vi "cache tag indices.vi"(8 "error in":errorcluster, 9 "index cluster":variant, 10 "channel classification":T1, 11 "fixed channel runtime in":refnum<class "user control module.lvclass">) -> (0 "error out":errorcluster, 3 "fixed channel runtime out":refnum<class "user control module.lvclass">)   [LabVIEW 2013, in "user control module.lvclass"]
uses:
  user control module.lvclass
  <vilib>/NI/Tag Bus Module Framework/channel/channel classification.ctl
  configuration/input data indices.ctl
  user control module.lvclass/user control module.ctl
  configuration/output data indices.ctl
  configuration/parameter data indices.ctl
  configuration/result data indices.ctl
  configuration/user control module configuration.lvclass
  <vilib>/NI/Configuration Framework/NISE_CEF_TreeControl.lvlib
  <vilib>/NI/Tag Bus Module Framework/channel/TBM channel.lvclass
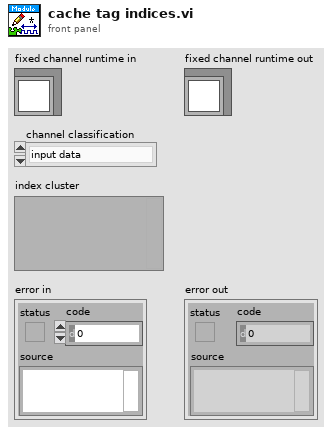
[diagram p1: front panel]
types:
  T1 = typedef "TBM channel.lvclass/channel classification.ctl" = enum16{"input data", "output data", "processing parameter", "processing result"}
  T2 = typedef "user control module configuration.lvclass/input data indices.ctl" = cluster{"Single.placeholder":i32}
  T3 = typedef "user control module configuration.lvclass/output data indices.ctl" = cluster{"Single.placeholder":i32}
  T4 = typedef "user control module configuration.lvclass/parameter data indices.ctl" = cluster{"Single.placeholder":i32}
  T5 = typedef "user control module configuration.lvclass/result data indices.ctl" = cluster{"Single.placeholder":i32}
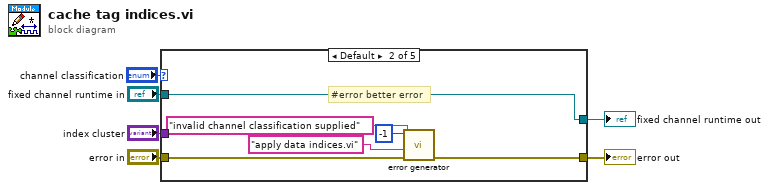
[diagram p0: block diagram]
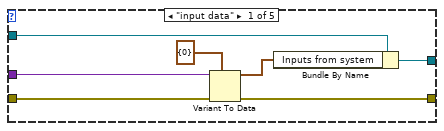
[diagram p2: hidden frame]
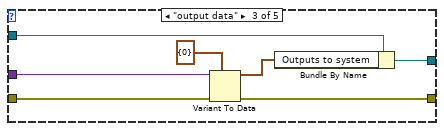
[diagram p3: hidden frame]
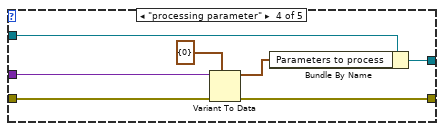
[diagram p4: hidden frame]
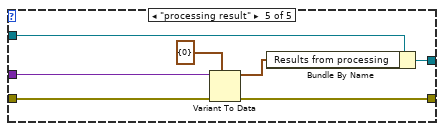
[diagram p5: hidden frame]
diagram:
  n1 = case shown="Default" "channel classification" {
    tunnel: "error in" -> [w11 w18 w24 w31 w38]
    tunnel: [w9 w17 w22 w29 w36] -> w5
    tunnel: [w12 w19 w25 w32 w39] -> w4
    tunnel: "fixed channel runtime in" -> [w13 w19 w26 w33 w40]
    tunnel: "index cluster" -> [w10 _ w23 w30 w37]
    frame "input data" {
      n2 = Variant To Data(error in=w11, type=T2 {"Single.placeholder"=0} ("Cluster"), Variant=w10) -> (data=w8:T2, error out=w9:errorcluster)
      n3 = Bundle By Name(cluster=w13, "Inputs from system"=w8) -> (w12:refnum<class "user control module.lvclass">)
    }
    frame Default {
      # "#error better error"
      n4 = call <vilib>:"error generator.vi"("error in"=w18, "source"="apply data indices.vi", "append error message"="invalid channel classification supplied", "error code (0)"=-1) -> ("error out"=w17:errorcluster)  [unwired: 5 in]
    }
    frame "output data" {
      n5 = Variant To Data(error in=w24, type=T3 {"Single.placeholder"=0} ("Cluster"), Variant=w23) -> (data=w21:T3, error out=w22:errorcluster)
      n6 = Bundle By Name(cluster=w26, "Outputs to system"=w21) -> (w25:refnum<class "user control module.lvclass">)
    }
    frame "processing parameter" {
      n7 = Variant To Data(error in=w31, type=T4 {"Single.placeholder"=0} ("Cluster"), Variant=w30) -> (data=w28:T4, error out=w29:errorcluster)
      n8 = Bundle By Name(cluster=w33, "Parameters to process"=w28) -> (w32:refnum<class "user control module.lvclass">)
    }
    frame "processing result" {
      n9 = Variant To Data(error in=w38, type=T5 {"Single.placeholder"=0} ("Cluster"), Variant=w37) -> (data=w35:T5, error out=w36:errorcluster)
      n10 = Bundle By Name(cluster=w40, "Results from processing"=w35) -> (w39:refnum<class "user control module.lvclass">)
    }
  }
  "error out" <- w5
  "fixed channel runtime out" <- w4
